vi "CAEN_HVBoard.constructor.vi"(0 "name":string, 2 "data in":string, 5 "error in(no error)":errorcluster) -> (14 "i ref out":refnum<vi>, 16 "data out":string, 19 "error out":errorcluster)   [LabVIEW 2014, in "CAEN_HVBoard.lvlib"]
doc: "This is the constructor of a class.\n\nLicense Agreement for this software:\n\nCopyright (C)\nGesellschaft für Schwerionenforschung, GSI\nPlanckstr. 1\n64291 Darmstadt\nGermany\n\nContact: D.Beck@gsi.de \n\nThis program is free software; you can redistribute it and/or modify it under the terms of the \nGNU General Public License as published by the Free Software Foundation; either version 2 of \nthe license, or (at your option) any later version.\n\nThis program is distributed in the hope that it will be useful, but WITHOUT ANY WARRANTY; \nwithout even the implied warranty of MERCHANTABILITY or FITNESS FOR A PARTICULAR PURPOSE. See the GNU General License for more details (http://www.gnu.org).\n\nGesellschaft für Schwerionenforschung, GSI\nPlanckstr. 1, 64291 Darmstadt, Germany\nFor all questions and ideas contact: M.Richter@gsi.de, H.Brand@gsi.de or D.Beck@gsi.de.\nLast update: 16-JUN-2004"
uses:
  CAEN_HVBoard.lvlib
  CAEN_HVBoard.i attribute.ctl
  CS_Core/CSApplicationBaseClasses/DeviceBase/DeviceBase.deviceState.ctl
  CS_Core/CSApplicationBaseClasses/DeviceBase/DeviceBase.myEventNames.ctl
  CS_Core/CSApplicationBaseClasses/DeviceBase/DeviceBase.lvlib
  CS_Core/CSSystem/CSSystemLib/CSSystemLib.lvlib
  CS_Core/BaseProcess/BaseProcess.lvlib
  CSlibraries-extern/DimLVEvent/LVDimInterface/LVDimInterface.lvlib
  CAEN_HVSystem/CAEN_HVSystem.lvlib
panel:
  in  "CLASS.i attribute":T1 {"BdStatus"."BdStatus" format="%.0b"; "Temp#Multiplier" format="%#.1e"; "HVMaxMultiplier" format="%#.1e"}
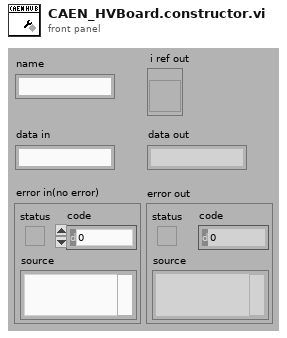
[diagram p1: front panel]
types:
  T1 = typedef "CAEN_HVBoard.lvlib/CAEN_HVBoard.i attribute.ctl" = cluster{"System Name":string, "Board ID":i32, "Prefix":string, "HVMaxMultiplier":dbl, "Temp#Multiplier":dbl, "Model Name":cluster{"Model Name":string, "DIM Status":cluster{"no link":bool, "quality":i32, "Time Stamp":timestamp}}, "Description":cluster{"Description":string, "DIM Status":cluster{"no link":bool, "quality":i32, "Time Stamp":timestamp}}, "SerNum":cluster{"SerNum":i16, "DIM Status":cluster{"no link":bool, "quality":i32, "Time Stamp":timestamp}}, "NrOfCh":cluster{"NrOfCh":i16, "DIM Status":cluster{"no link":bool, "quality":i32, "Time Stamp":timestamp}}, "BdStatus":cluster{"BdStatus":i16, "DIM Status":cluster{"no link":bool, "quality":i32, "Time Stamp":timestamp}}, "HVMax":cluster{"HVMax":dbl, "DIM Status":cluster{"no link":bool, "quality":i32, "Time Stamp":timestamp}}, "HVMax#EU":cluster{"HVMax#EU":string, "DIM Status":cluster{"no link":bool, "quality":i32, "Time Stamp":timestamp}}, "HVMax#HighEU":cluster{"HVMax#HighEU":dbl, "DIM Status":cluster{"no link":bool, "quality":i32, "Time Stamp":timestamp}}, "HVMax#LowEU":cluster{"HVMax#LowEU":dbl, "DIM Status":cluster{"no link":bool, "quality":i32, "Time Stamp":timestamp}}, "Temp#EU":cluster{"Temp#EU":string, "DIM Status":cluster{"no link":bool, "quality":i32, "Time Stamp":timestamp}}, "Temp":cluster{"Temp":dbl, "DIM Status":cluster{"no link":bool, "quality":i32, "Time Stamp":timestamp}}, "Temp#HighEU":cluster{"Temp#HighEU":dbl, "DIM Status":cluster{"no link":bool, "quality":i32, "Time Stamp":timestamp}}, "Temp#LowEU":cluster{"Temp#LowEU":dbl, "DIM Status":cluster{"no link":bool, "quality":i32, "Time Stamp":timestamp}}}
  T2 = enum16{"SetAttribute", "GetAttribute", "CreateAttribute", "DestroyAttribute", "DestroyAllAtributes"}
  T3 = typedef "DeviceBase.lvlib/DeviceBase.myEventNames.ctl" = enum16{"lvmsg://Initialize", "lvmsg://Close", "lvmsg://Configure", "lvmsg://Reset", "lvmsg://IDQuery"}
  T4 = typedef "DeviceBase.lvlib/DeviceBase.deviceState.ctl" = i16
  T5 = typedef "BaseProcess.lvlib/BaseProcess.i attribute.ctl" = cluster{"EventStatus":string, "EventError":i32, "PresetEvtWatchD":i32, "PresetPdcWatchD":i32, "EventTimeout":i32, "PeriodicInterval":i32, "Interface":string[], "Address":string[], "Special":string[], "PeriodicError":i32, "PeriodicStatus":string, "SuperProc":string, "Descriptors":T6[], "CaseRef":refnum<vi>, "PdcRef":refnum<vi>, "Thread Ref":refnum<vi>, "eventErrorID":i32, "eventStatusID":i32, "periodicErrorID":i32, "periodicStatusID":i32, "pdcCtrID":i32}
  T6 = typedef "BaseProcess.lvlib/BaseProcess.descriptor definition.ctl" = cluster{"selector":string, "descriptor":T7}
  T7 = typedef "BaseProcess.lvlib/BaseProcess.descriptor string definition.ctl" = string
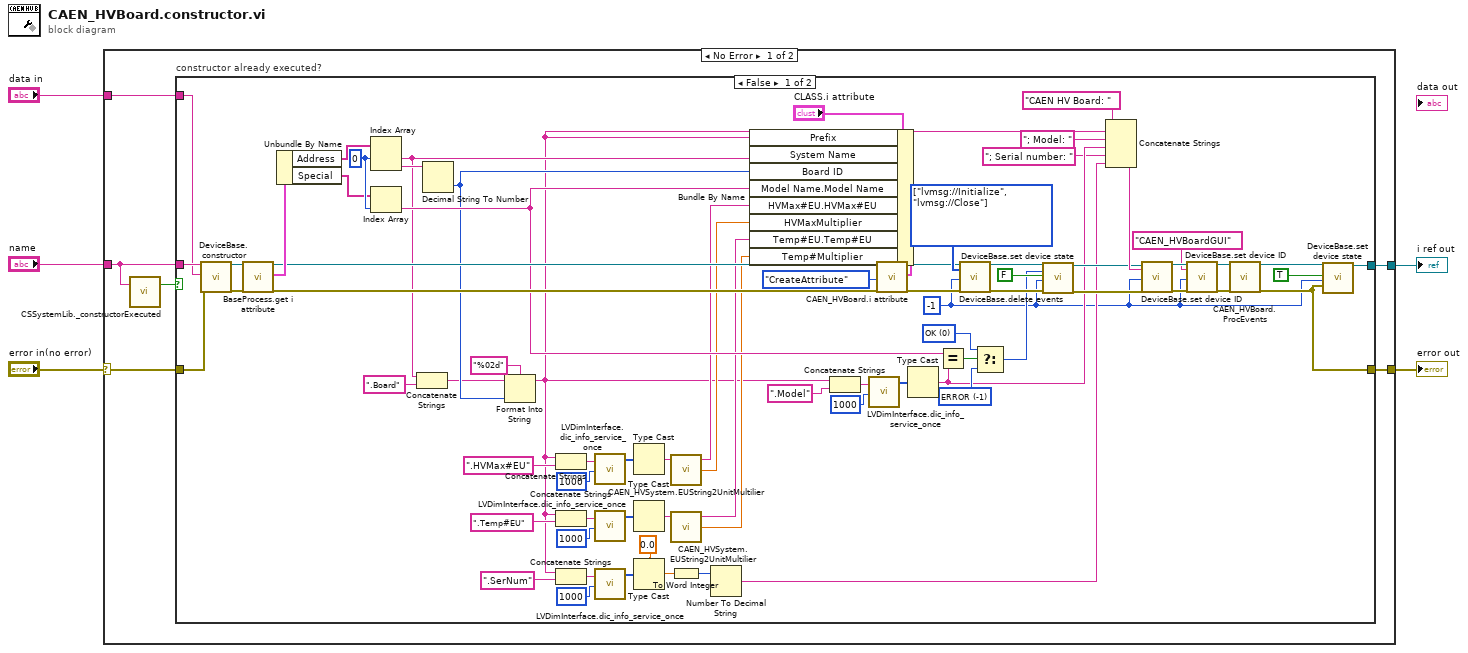
[diagram p0: block diagram]
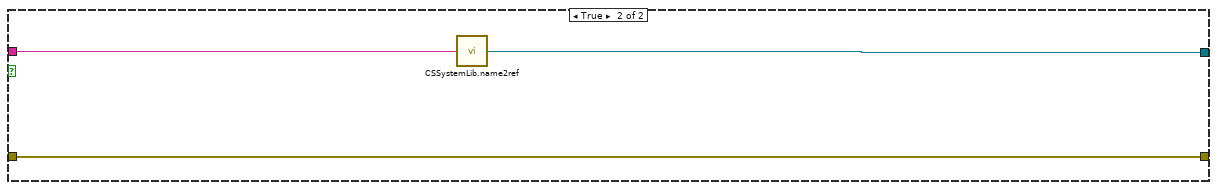
[diagram p2: hidden frame]
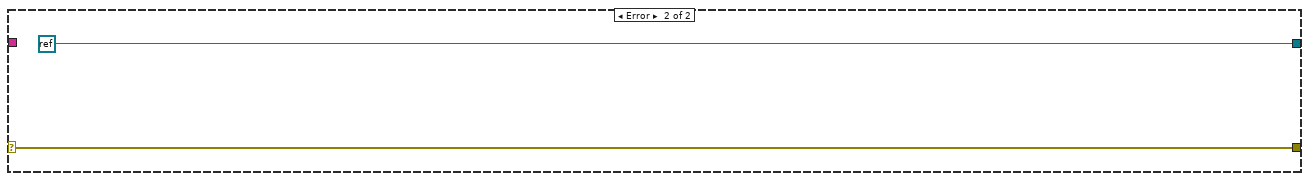
[diagram p3: hidden frame]
diagram:
  n1 = case shown="No Error" "error in(no error)" {
    selector: "error in(no error)" -> [w9 w90]
    tunnel: "name" -> [w8 _]
    tunnel: [w11 refnum<k0> refnum] -> w4
    tunnel: [w10 w90] -> w3
    tunnel: "data in" -> [w6 _]
    frame No Error {
      n2 = call "CSSystemLib._constructorExecuted.vi"("name"=w8) -> ("constructor executed?"=w7:bool)  [unwired: 18 in]
      n3 = case "constructor already executed?" shown="False" w7 {
        tunnel: w8 -> [w85 w89]
        tunnel: [w73 w88] -> w11
        tunnel: [w42 w87] -> w10
        tunnel: w9 -> [w84 w87]
        tunnel: w6 -> [w83 _]
        frame False {
          w74 = T3[] [enum."lvmsg://Initialize", enum."lvmsg://Close"] items=["lvmsg://Initialize", "lvmsg://Close", "lvmsg://Configure", "lvmsg://Reset", "lvmsg://IDQuery"] ("events")
          w61 = T4 -1 items=["ERROR"=-1, "OK"=0, "NOT_OK"=1] ("deviceState")
          w57 = T4 0 items=["ERROR"=-1, "OK"=0, "NOT_OK"=1] ("deviceState")
          w72 = 0 ("index")
          w13 = -1 ("ms timeout (10000)")
          n4 = call "DeviceBase.constructor.vi"("name"=w85, "data in"=w83, "error in (no error)"=w84) -> ("i ref out"=w67:refnum<vi>, "error out"=w68:errorcluster)  [unwired: 14 in, 1 out]
          n5 = call "BaseProcess.get i attribute.vi"("i ref in"=w67, "error in (no error)"=w68) -> ("i ref out"=w66:refnum<vi>, "i attribute"=w69:T5, "error out"=w65:errorcluster)  [unwired: 15 in]
          n6 = Unbundle By Name(w69) -> ("Address"=w70:string[], "Special"=w71:string[])
          n7 = Index Array(array=w70, index #1=w72) -> (element #1=w48:string, element #2=w62:string)  [unwired: 1 in]
          n8 = Index Array(array=w71, index=w72) -> (element=w54:string)
          n9 = Concatenate Strings(w48, ".Board" ("format string")) -> (w47:string)
          n10 = Decimal String To Number(string=w62) -> (number=w53:i32)  [unwired: 2 in, 1 out]
          n11 = Format Into String(format string="%02d", initial string=w47, w53) -> (resulting string=w18:string)  [unwired: 1 in, 1 out]
          n12 = Concatenate Strings(w18, ".HVMax#EU" ("string")) -> (w41:string)
          n13 = Concatenate Strings(w18, ".Temp#EU" ("string")) -> (w34:string)
          n14 = Concatenate Strings(w18, ".SerNum" ("string")) -> (w27:string)
          n15 = call "LVDimInterface.dic_info_service_once.vi"("serviceName"=w41, "timeout [ms]"=u32 1000) -> ("data"=w38:i8[])  [unwired: 14 in, 3 out]
          n16 = call "LVDimInterface.dic_info_service_once.vi"("serviceName"=w34, "timeout [ms]"=u32 1000) -> ("data"=w37:i8[])  [unwired: 14 in, 3 out]
          n17 = call "LVDimInterface.dic_info_service_once.vi"("serviceName"=w27, "timeout [ms]"=u32 1000) -> ("data"=w24:i8[])  [unwired: 14 in, 3 out]
          n18 = Type Cast(x=w38) -> (*(type *) &x=w33:string)  [unwired: 1 in]
          n19 = Type Cast(x=w37) -> (*(type *) &x=w32:string)  [unwired: 1 in]
          n20 = Type Cast(type=0.0, x=w24) -> (*(type *) &x=w21:dbl)
          n21 = call "CAEN_HVSystem.EUString2UnitMultilier.vi"("EU String"=w33) -> ("Multiplier"=w31:dbl, "Unit"=w29:string)  [unwired: 2 in, 1 out]
          n22 = call "CAEN_HVSystem.EUString2UnitMultilier.vi"("EU String"=w32) -> ("Multiplier"=w30:dbl, "Unit"=w28:string)  [unwired: 2 in, 1 out]
          n23 = To Word Integer(number=w21) -> (16bit integer=w20:i16)
          n24 = Number To Decimal String(number=w20) -> (decimal integer string=w19:string)  [unwired: 1 in]
          n25 = Bundle By Name(cluster="CLASS.i attribute", "Prefix"=w18, "System Name"=w48, "Board ID"=w53, "Model Name.Model Name"=w54, "HVMax#EU.HVMax#EU"=w29, "HVMaxMultiplier"=w31, "Temp#EU.Temp#EU"=w28, "Temp#Multiplier"=w30) -> (w63:T1)
          n26 = Concatenate Strings(w18, ".Model" ("string")) -> (w50:string)
          n27 = call "LVDimInterface.dic_info_service_once.vi"("serviceName"=w50, "timeout [ms]"=u32 1000) -> ("data"=w59:i8[])  [unwired: 14 in, 3 out]
          n28 = call "CAEN_HVBoard.i attribute.vi"("VI Refnum"=w66, "CLASS.i attribute"=w63, "Action"=T2."CreateAttribute", "error in (no error)"=w65) -> ("VI Refnum out"=w45:refnum<vi>, "error out"=w44:errorcluster)  [unwired: 13 in, 1 out]
          n29 = Type Cast(x=w59) -> (*(type *) &x=w55:string)  [unwired: 1 in]
          n30 = Equal?(x=w54, y=w55) -> (x = y?=w60:bool)
          n31 = call "DeviceBase.delete events.vi"("i ref in"=w45, "events"=w74, "ms timeout (10000)"=w13, "error in (no error)"=w44) -> ("i ref out"=w77:refnum<vi>, "error out"=w76:errorcluster)  [unwired: 13 in, 1 out]
          n32 = Select(t=w57, s=w60, f=w61) -> (s? t:f=w56:T4)
          n33 = call "DeviceBase.set device state.vi"("i ref in"=w77, "deviceState"=w56, "implicit"=FALSE, "ms timeout (10000)"=w13, "error in (no error)"=w76) -> ("i ref out"=w78:refnum<vi>, "error out"=w79:errorcluster)  [unwired: 12 in, 1 out]
          n34 = Concatenate Strings("CAEN HV Board: " ("string"), w18, "; Model: " ("string"), w55, "; Serial number: " ("string"), w19) -> (w82:string)
          n35 = call "DeviceBase.set device ID.vi"("i ref in"=w78, "deviceID"=w82, "ms timeout (10000)"=w13, "error in (no error)"=w79) -> ("i ref out"=w17:refnum<vi>, "error out"=w15:errorcluster)  [unwired: 13 in, 1 out]
          n36 = call "DeviceBase.set device ID.vi"("i ref in"=w17, "deviceID"="CAEN_HVBoardGUI", "ms timeout (10000)"=w13, "error in (no error)"=w15) -> ("i ref out"=w16:refnum<vi>, "error out"=w14:errorcluster)  [unwired: 13 in, 1 out]
          n37 = call "CAEN_HVBoard.ProcEvents.vi"("i ref in"=w16, "error in"=w14) -> ("i ref out"=w43:refnum<vi>, "error out"=w42:errorcluster)  [unwired: 16 in]
          n38 = call "DeviceBase.set device state.vi"("i ref in"=w43, "implicit"=TRUE, "ms timeout (10000)"=w13, "device error"=w42) -> ("i ref out"=w73:refnum<vi>)  [unwired: 13 in, 2 out]
        }
        frame True {
          n39 = call "CSSystemLib.name2ref.vi"("name"=w89) -> ("obj refnum"=w88:refnum<vi>)
        }
      }
    }
    frame Error {
    }
  }
  "i ref out" <- w4
  "error out" <- w3
